vi "DirettorePlay.vi"(0 "FPGAReference":refnum<k20>, 1 "NumberOfMatrices":i32, 5 "MatricesArray":i16[](array[numeric]), 7 "DeltaTimeArray":i32[](array[numeric]), 9 "NumberOfTimePointsToPlayArray":i32[](array[numeric]), 11 "SyncArray":i32[](array[numeric])) -> (4 "SpaceLeftInQueue":u32, 15 "ErrorOut":errorcluster)   [LabVIEW 2012]
uses:
  <vilib>/Utility/error.llb/Error Cluster From Error Code.vi
  <vilib>/rvi/errors/niLvFpgaAdjustHostInterfaceError.vi
  <vilib>/rvi/interface/nirviMethod/nirviMethod.xnode
  <vilib>/FPGAPlugInAG/Dynamic/niLvFpga_WriteFifo_Dynamic.vi
  <vilib>/rvi/errors/niLvFpgaMergeErrorWithErrorCode.vi
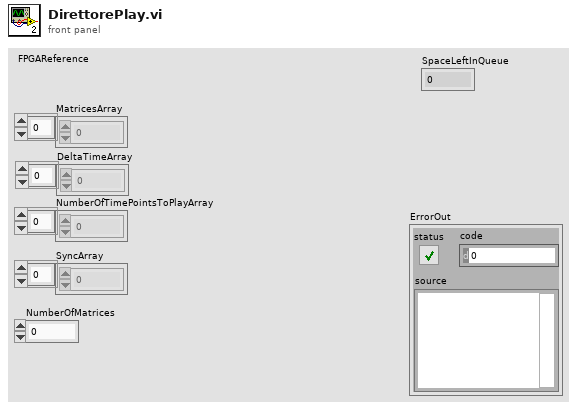
[diagram p1: front panel]
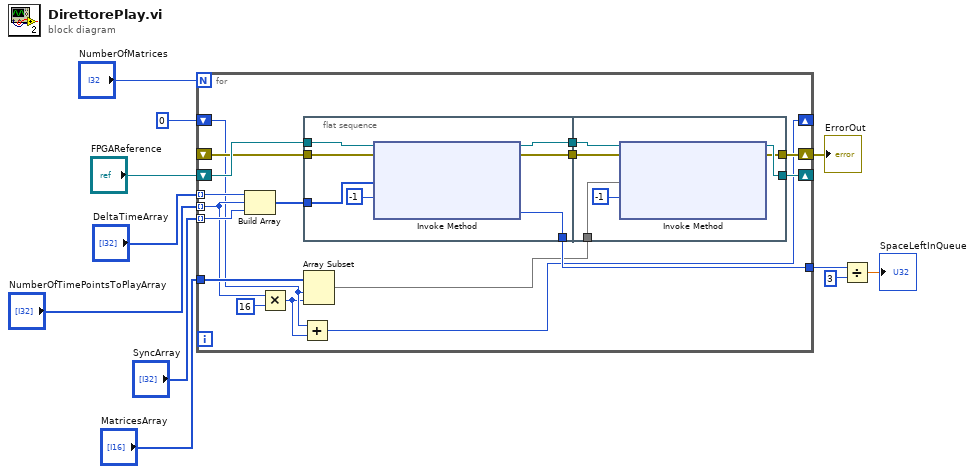
[diagram p0: block diagram]
diagram:
  n1 = for {
    N: "NumberOfMatrices" -> [_]
    shift-right: [w26] -> _
    shift-left: "FPGAReference" -> [w28]
    shift-right: [w25] -> w11
    shift-left: _ -> [w27]
    tunnel: "SyncArray" -> [w20] mode=indexing
    tunnel: "DeltaTimeArray" -> [w21] mode=indexing
    tunnel: [w19] -> w5
    tunnel: "NumberOfTimePointsToPlayArray" -> [w16] mode=indexing
    tunnel: "MatricesArray" -> [w17]
    shift-right: [w13] -> _
    shift-left: 0 ("index") -> [w14]
    n2 = Build Array(w21, w16, w20) -> (w24:i32[])
    n3 = Multiply(x=w16, y=16) -> (x*y=w12:i32)
    n4 = Add(x=w14, y=w12) -> (x+y=w13:i32)
    n5 = flat-sequence {
      tunnel: w28 -> [w34]
      tunnel: w27 -> [w33]
      tunnel: w24 -> [w32]
      tunnel: [w31] -> w23
      tunnel: [w30] -> w22
      tunnel: [w29] -> w19
      tunnel: w18 -> [w38]
      tunnel: [w40] -> w26
      tunnel: [w39] -> w25
      tunnel: w23 -> [w37]
      tunnel: w22 -> [w36]
      frame #0 {
        n6 = xnode "Invoke Method"("FPGA VI Reference In"=w34, "error in"=w33, "Data"=w32, "Timeout (ms)"=-1) -> ("FPGA VI Reference Out"=w31:refnum<k20>, "error out"=w30:errorcluster, "Empty Elements Remaining"=w29:u32)
      }
      frame #1 {
        n7 = xnode "Invoke Method"("FPGA VI Reference In"=w37, "error in"=w36, "Data"=w38, "Timeout (ms)"=-1) -> ("FPGA VI Reference Out"=w40:refnum<k20>, "error out"=w39:errorcluster)  [unwired: 1 out]
      }
    }
    n8 = Array Subset(array=w17, index=w14, length=w12) -> (w18:i16[])
  }
  "ErrorOut" <- w11
  n9 = Divide(x=w5, y=u32 3) -> (x/y=→"SpaceLeftInQueue":dbl)
